vi "5.1.vi"() -> ()   [LabVIEW 2022 SP3]
panel:
  out "Square with Uniform Noise":dynamicdata(graph)
  # "Aditya Singh"
  # "2315005"
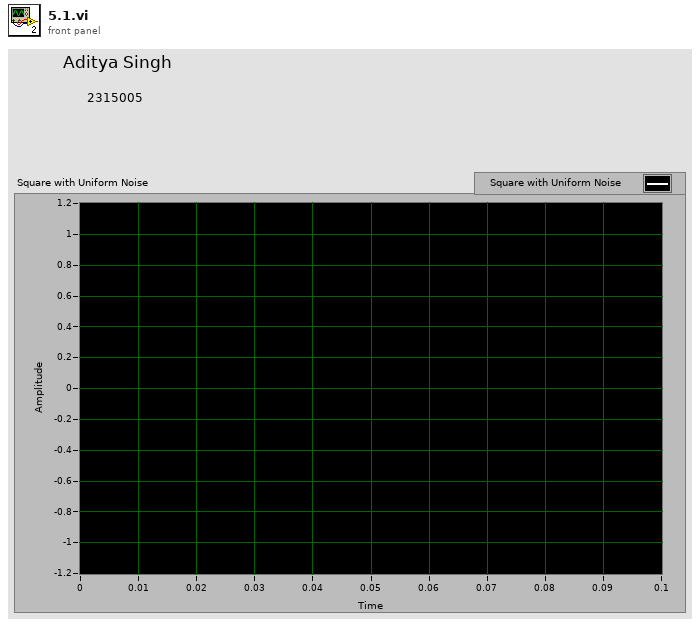
[diagram p1: front panel]
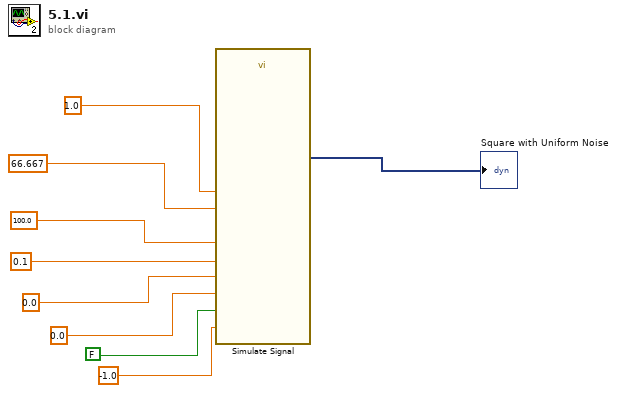
[diagram p0: block diagram]
diagram:
  n1 = call "Simulate Signal"("Offset"=0.0, "Duty Cycle (%)"=66.667, "Reset Signal"=FALSE, "Frequency"=100.0, "Amplitude"=1.0, "Phase"=0.0, "Noise amplitude"=0.1, "Seed Number"=-1.0) -> ("Square with Uniform Noise"=→"Square with Uniform Noise":dynamicdata)  [unwired: 6 in, 1 out]
